vi "Create Websockets Connection.vi"(5 "WSConnection in":refnum<class "WebsocketsConnection.lvclass">, 8 "error in (no error)":errorcluster, 11 "WebSocket":refnum<class "WebSocket.lvclass">) -> (0 "error out":errorcluster, 3 "WSConnection":refnum<class "WebsocketsConnection.lvclass">)   [LabVIEW 2013, in "MQTT_Websockets.lvlib" / "WebsocketsConnection.lvclass"]
uses:
  WebsocketsConnection.lvclass
  <vilib>/MediaMongrels Ltd/WebSockets/WebSockets/WebSocket/WebSocket.lvclass
  WebsocketsConnection.lvclass/WebsocketsConnection.ctl
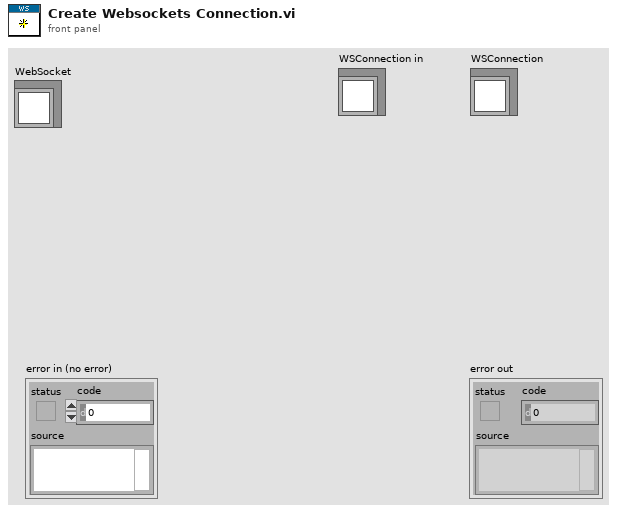
[diagram p1: front panel]
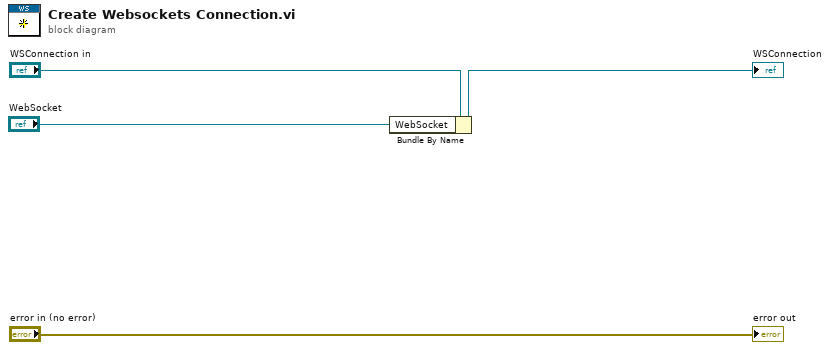
[diagram p0: block diagram]
diagram:
  n1 = Bundle By Name(cluster="WSConnection in", "WebSocket"="WebSocket") -> (→"WSConnection":refnum<class "WebsocketsConnection.lvclass">)
  "error out" <- "error in (no error)"
